vi "BinarySearch.vi"(2 "value searching for":dbl format="%0.2f", 3 "Sorted Array":dbl[](array[numeric])) -> (0 "index":i32, 1 "isFound":bool)   [LabVIEW 2017, in "NI_PtbyPt.lvlib"]
uses:
  <vilib>/ptbypt/NI_PtbyPt.lvlib
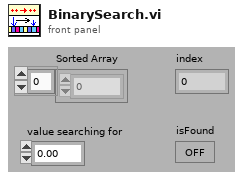
[diagram p1: front panel]
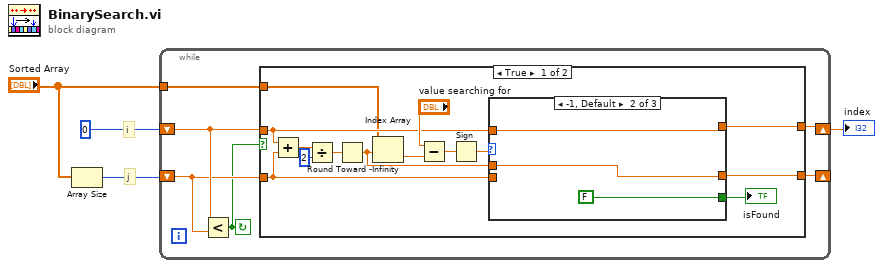
[diagram p0: block diagram]
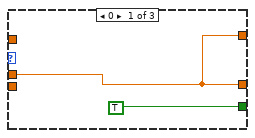
[diagram p2: hidden frame]
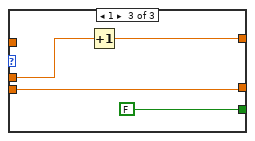
[diagram p3: hidden frame]
diagram:
  # "j"
  # "i"
  n1 = Array Size(array="Sorted Array") -> (size(s)=w3:i32)
  n2 = while {
    tunnel: "Sorted Array" -> [w5]
    shift-left: w3 -> [w7]
    shift-right: [w9] -> _
    shift-left: 0 -> [w8]
    shift-right: [w10] -> w2
    stop <- w6 continue-if-true
    n3 = Less?(x=w8, y=w7) -> (x < y?=w6:bool)
    n4 = case shown="True" w6 {
      tunnel: [w16 w35] -> w10
      tunnel: [w15 w34] -> w9
      tunnel: w8 -> [w14 w35]
      tunnel: w7 -> [w13 w34]
      tunnel: w5 -> [w12 _]
      frame True {
        n5 = Add(x=w14, y=w13) -> (x+y=w23:dbl)
        n6 = Divide(x=w23, y=2) -> (x/y=w22:dbl)
        n7 = Round Toward -Infinity(1:w22) -> (0:w17:dbl)
        n8 = Index Array(array=w12, index=w17) -> (element=w20:dbl)
        n9 = Subtract(x="value searching for", y=w20) -> (x-y=w19:dbl)
        n10 = Sign(1:w19) -> (0:w18:dbl)
        n11 = case shown="-1, Default" w18 {
          tunnel: w17 -> [w26 w29 w33]
          tunnel: [w26 w28 w30] -> w16
          tunnel: [w26 w29 w32] -> w15
          tunnel: w14 -> [_ w28 _]
          tunnel: w13 -> [_ _ w32]
          tunnel: [TRUE ("isFound") FALSE ("isFound") FALSE ("isFound")] -> w11
          frame 0 {
          }
          frame -1, Default {
          }
          frame 1 {
            n12 = Increment(x=w33) -> (x+1=w30:dbl)
          }
        }
        "isFound" <- w11
      }
      frame False {
      }
    }
  }
  "index" <- w2
